vi "TurnDistanceAuto.vi"(8 "error in":errorcluster, 9 "Timeout":dbl, 10 "Degrees":dbl, 11 "MaxSpeed":dbl) -> (0 "error out":errorcluster, 3 "Done":bool)   [LabVIEW 2020]
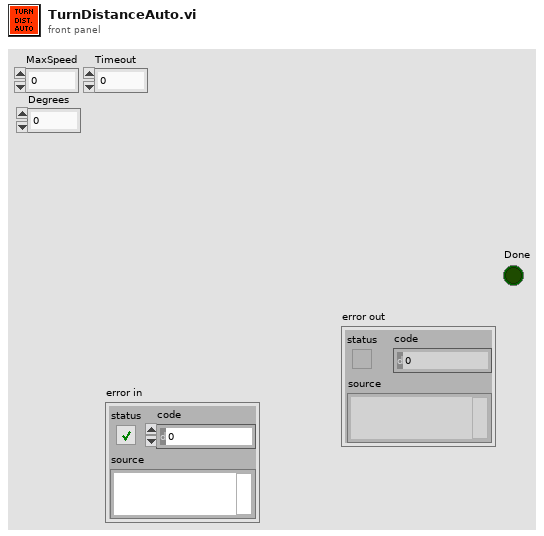
[diagram p1: front panel]
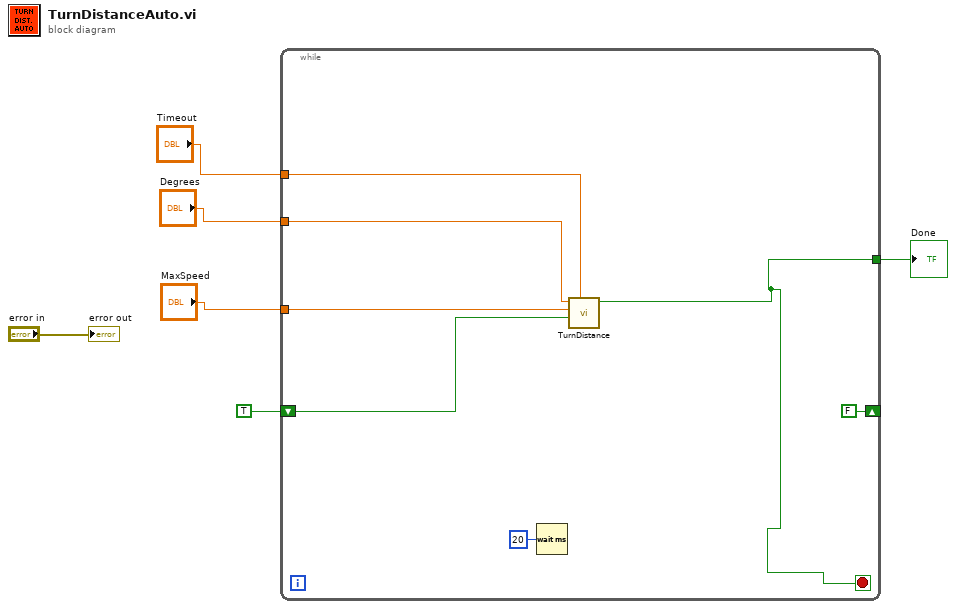
[diagram p0: block diagram]
diagram:
  n1 = while {
    tunnel: [w8] -> w5
    tunnel: "MaxSpeed" -> [w10]
    tunnel: "Degrees" -> [w11]
    tunnel: "Timeout" -> [w12]
    shift-right: [FALSE] -> _
    shift-left: TRUE -> [w9]
    stop <- w8 stop-if-true
    n2 = Wait (ms)(milliseconds to wait=u32 20) -> ()  [unwired: 1 out]
    n3 = call "TurnDistance.vi"("Timeout"=w12, "Initation?"=w9, "MaxSpeed"=w10, "Degrees"=w11) -> ("Finished"=w8:bool)  [unwired: 5 in, 2 out]
  }
  "Done" <- w5
  "error out" <- "error in"
